vi "power conversion.vi"(8 "error in (no error)":errorcluster, 11 "AOTF in":refnum<class "AOTF.lvclass">) -> (0 "error out":errorcluster, 2 "Power voltage out":dbl, 3 "AOTF out":refnum<class "AOTF.lvclass">)   [LabVIEW 2012, in "AOTF.lvclass"]
uses:
  AOTF.lvclass
  AOTF.lvclass/AOTF.ctl
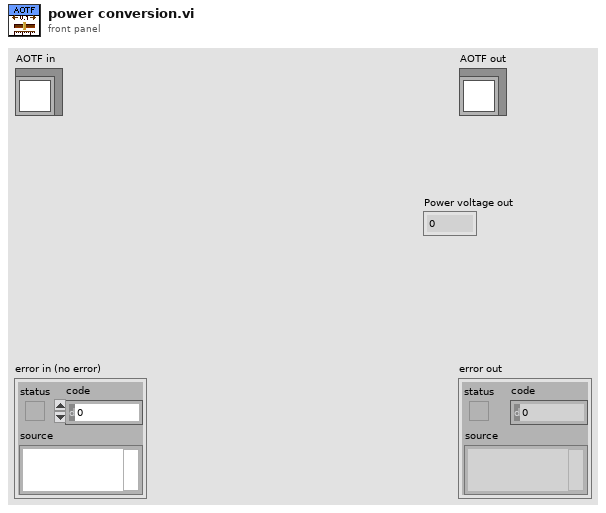
[diagram p1: front panel]
types:
  T1 = typedef "AOTF.lvclass/laser line ring.ctl" = u8
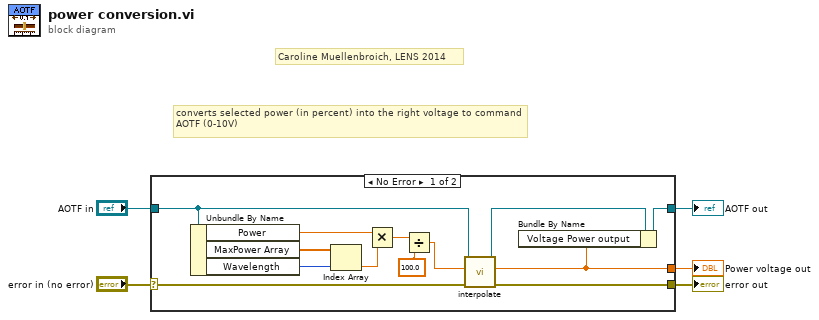
[diagram p0: block diagram]
diagram:
  # "converts selected power (in percent) into the right voltage to command AOTF (0-10V)"
  # "Caroline Muellenbroich, LENS 2014"
  n1 = case shown="No Error" "error in (no error)" {
    selector: "error in (no error)" -> [w18 w20]
    tunnel: [w17 w20] -> w4
    tunnel: [w7 w19] -> w2
    tunnel: "AOTF in" -> [w10 w19]
    tunnel: [w6 _] -> w1
    frame No Error {
      n2 = Unbundle By Name(w10) -> ("Power"=w16:dbl, "MaxPower Array"=w13:dbl[], "Wavelength"=w12:T1)
      n3 = Index Array(array=w13, index=w12) -> (element=w11:dbl)
      n4 = Multiply(x=w16, y=w11) -> (x*y=w15:dbl)
      n5 = Divide(x=w15, y=100.0) -> (x/y=w9:dbl)
      n6 = call-dynamic "interpolate.vi"("error in (no error)"=w18, "Power in"=w9, "AOTF in"=w10) -> ("error out"=w17:errorcluster, "Power voltage out"=w6:dbl, "AOTF out"=w8:refnum<class "AOTF.lvclass">)  [unwired: 6 in]
      n7 = Bundle By Name(cluster=w8, "Voltage Power output"=w6) -> (w7:refnum<class "AOTF.lvclass">)
    }
    frame Error {
    }
  }
  "error out" <- w4
  "AOTF out" <- w2
  "Power voltage out" <- w1
